vi "RD Analog In Trigger Level Set.vi"(8 "error in (no error)":errorcluster caption="错误输入（无错误）", 9 "range":i32=5, 10 "voltsLevel":dbl, 11 "handle":u64) -> (0 "error out":errorcluster caption="错误输出", 2 "function return":i32, 3 "handle out":u64)   [LabVIEW 2018, in "InstrumentsPlayground.lvlib"]
doc: "CLIFFAPI int CliffAnalogInTriggerLevelSet(FT_HANDLE handle, double voltsLevel);\nvoltsLevel: -5~5V or -25~25V"
uses:
  InstrumentsPlayground.lvlib
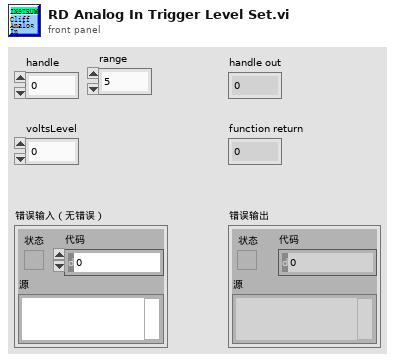
[diagram p1: front panel]
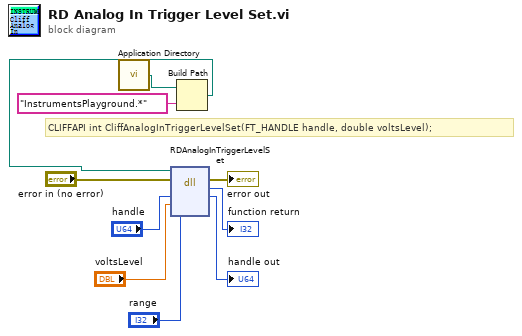
[diagram p0: block diagram]
diagram:
  # "CLIFFAPI int CliffAnalogInTriggerLevelSet(FT_HANDLE handle, double voltsLevel);"
  n1 = call <vilib>:"Application Directory.vi"() -> ("Application Directory"=w3:path)
  n2 = Build Path(base path=w3, name or relative path="InstrumentsPlayground.*" ("名称或相对路径")) -> (appended path=w2:path)
  n3 = dll-call lib="E:/work/YZCourse_Xtext/Cliff/API/LabVIEW lib/InstrumentsPlayground.*" fn="RDAnalogInTriggerLevelSet"(path in=w2, error in="error in (no error)", "handle"="handle", "voltsLevel"="voltsLevel", "range"="range") -> (error out=→"error out":errorcluster, "返回类型"=→"function return":i32, "handle"=→"handle out":u64)  [unwired: 3 in, 1 out]
